vi "RT_main.vi"() -> ()   [LabVIEW 2018]
panel:
  in  "set pos":bool
  in  "stop":bool
  in  "setpoint":i16(slide) scale=-1500.0..1500.0
  out "dt":u32
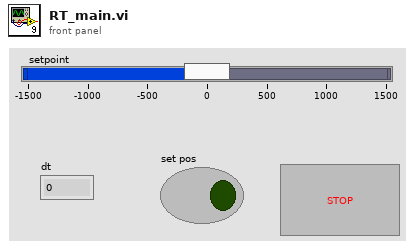
[diagram p1: front panel]
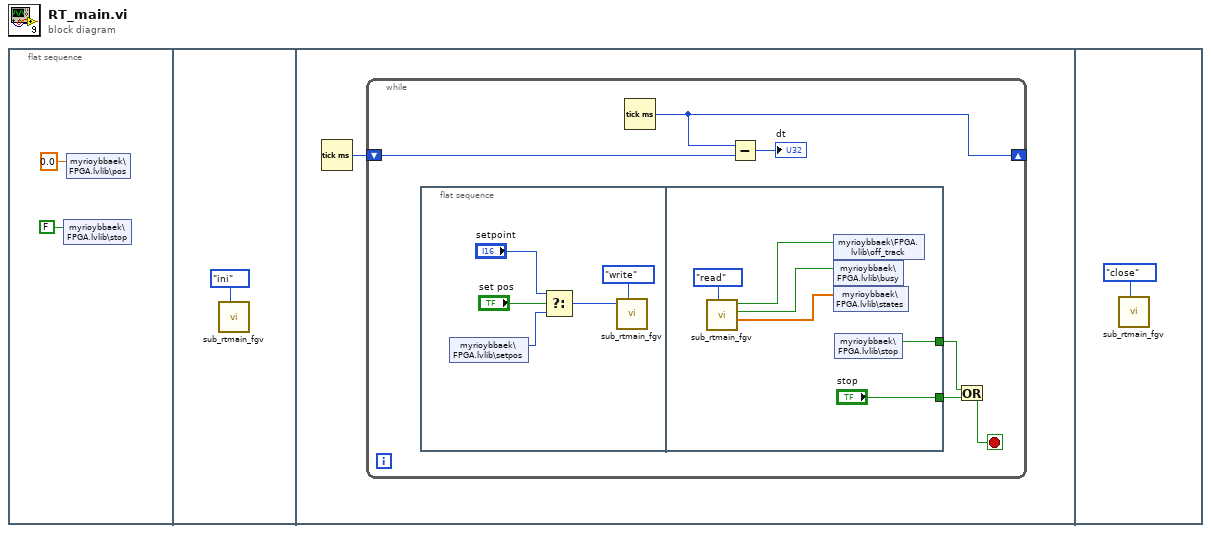
[diagram p0: block diagram]
diagram:
  n1 = flat-sequence {
    frame #0 {
      n2 = shared-variable "myrioybbaek\\FPGA.lvlib\\stop"(FALSE ("stop")) -> ()  [unwired: 1 in, 1 out]
      n3 = shared-variable "myrioybbaek\\FPGA.lvlib\\pos"(0.0 ("pos")) -> ()  [unwired: 1 in, 1 out]
    }
    frame #1 {
      n4 = call "sub_rtmain_fgv.vi"("cmd"=enum16{"ini", "read", "write", "close"}."ini") -> ()  [unwired: 7 in, 4 out]
    }
    frame #2 {
      n5 = Tick Count (ms)() -> (millisecond timer value=w4:u32)
      n6 = while {
        shift-right: [w10] -> _
        shift-left: w4 -> [w9]
        stop <- w5 stop-if-true
        n7 = flat-sequence {
          tunnel: [w21] -> w7
          tunnel: ["stop"] -> w6
          frame #0 {
            n8 = shared-variable "myrioybbaek\\FPGA.lvlib\\setpos"() -> (w11:i16)  [unwired: 1 in, 1 out]
            n9 = Select(t="setpoint", s="set pos", f=w11) -> (s? t:f=w12:i16)
            n10 = call "sub_rtmain_fgv.vi"("cmd"=enum16{"ini", "read", "write", "close"}."write", "setpoint"=w12) -> ()  [unwired: 6 in, 4 out]
          }
          frame #1 {
            n11 = call "sub_rtmain_fgv.vi"("cmd"=enum16{"ini", "read", "write", "close"}."read") -> ("states"=w20:dbl[], "busy"=w18:bool, "off_track"=w17:bool)  [unwired: 7 in, 1 out]
            n12 = shared-variable "myrioybbaek\\FPGA.lvlib\\off_track"(w17) -> ()  [unwired: 1 in, 1 out]
            n13 = shared-variable "myrioybbaek\\FPGA.lvlib\\busy"(w18) -> ()  [unwired: 1 in, 1 out]
            n14 = shared-variable "myrioybbaek\\FPGA.lvlib\\states"(w20) -> ()  [unwired: 1 in, 1 out]
            n15 = shared-variable "myrioybbaek\\FPGA.lvlib\\stop"() -> (w21:bool)  [unwired: 1 in, 1 out]
          }
        }
        n16 = Tick Count (ms)() -> (millisecond timer value=w10:u32)
        n17 = Subtract(x=w10, y=w9) -> (x-y=→"dt":u32)
        n18 = Or(x=w7, y=w6) -> (x .or. y?=w5:bool)
      }
    }
    frame #3 {
      n19 = call "sub_rtmain_fgv.vi"("cmd"=enum16{"ini", "read", "write", "close"}."close") -> ()  [unwired: 7 in, 4 out]
    }
  }
